vi "Map-characteristics.vi"(8 "error in (no error)":errorcluster, 11 "Data ref. in":refnum<data-value>) -> (0 "error out":errorcluster, 3 "Data ref.":refnum<data-value>)   [LabVIEW 2013, in "CameraVision.lvlib" / "CV-Main.lvclass"]
uses:
  CV-Main.lvclass
  Buffers/Mapping-buffer.ctl
  Temperature/Temperature-characteristics.ctl
  Analysis/Characteristics-cluster.ctl
  CV-Main.lvclass/CV-Main.ctl
  Buffers/CV-Buffers.lvclass/CV-Buffers.ctl
  Mapping/CV-Mapping.lvclass/CV-Mapping.ctl
  Read Buffers.vi
  Read Mapping params.vi
  Read Map.vi
  Read Processing.vi
  Mapping/Read Time.vi
  Mapping/Read Xcoors.vi
  Mapping/Read Ycoors.vi
  Mapping/Read Enable mapping.vi
  Buffers/Read Mapping buffer.vi
  Buffers/CV-Buffers.lvclass
  Mapping/CV-Mapping.lvclass
  UI/CV-UI.lvclass
  Temperature/CV-Temperature.lvclass
  Analysis/CV-Analysis.lvclass
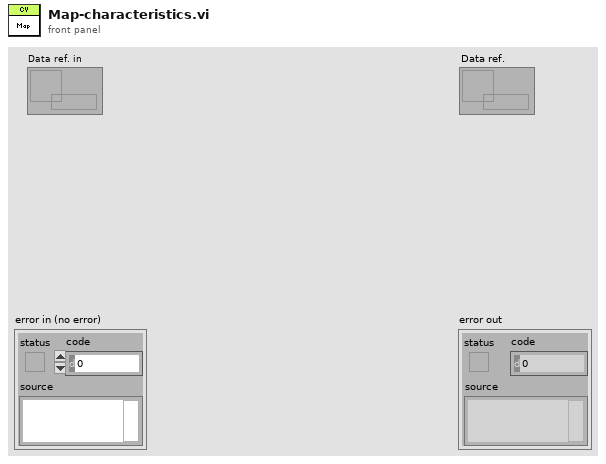
[diagram p1: front panel]
types:
  T1 = typedef "CameraVision.lvlib/CV-Buffers.lvclass/Mapping-buffer.ctl" = cluster{"Time":timestamp, "Index":i32, "Temperature characteristics":T2, "Characteristics":T3[], "Xcoord":sgl, "Ycoord":sgl}
  T2 = typedef "CameraVision.lvlib/CV-Temperature.lvclass/Temperature-characteristics.ctl" = cluster{"Average temperature ":dbl, "Max. temperature":dbl, "Min. temperature":dbl, "Stand. dev. temperature":dbl, "Datapoints":dbl}
  T3 = typedef "CameraVision.lvlib/CV-Analysis.lvclass/Characteristics-cluster.ctl" = cluster{"Average intensity":dbl, "Peak intensity":dbl, "Melt-pool size":dbl, "Melt-pool aspect ratio":dbl, "Melt-pool fragments":dbl, "Centre of mass X":dbl, "Centre of mass Y":dbl, "Orientation":dbl}
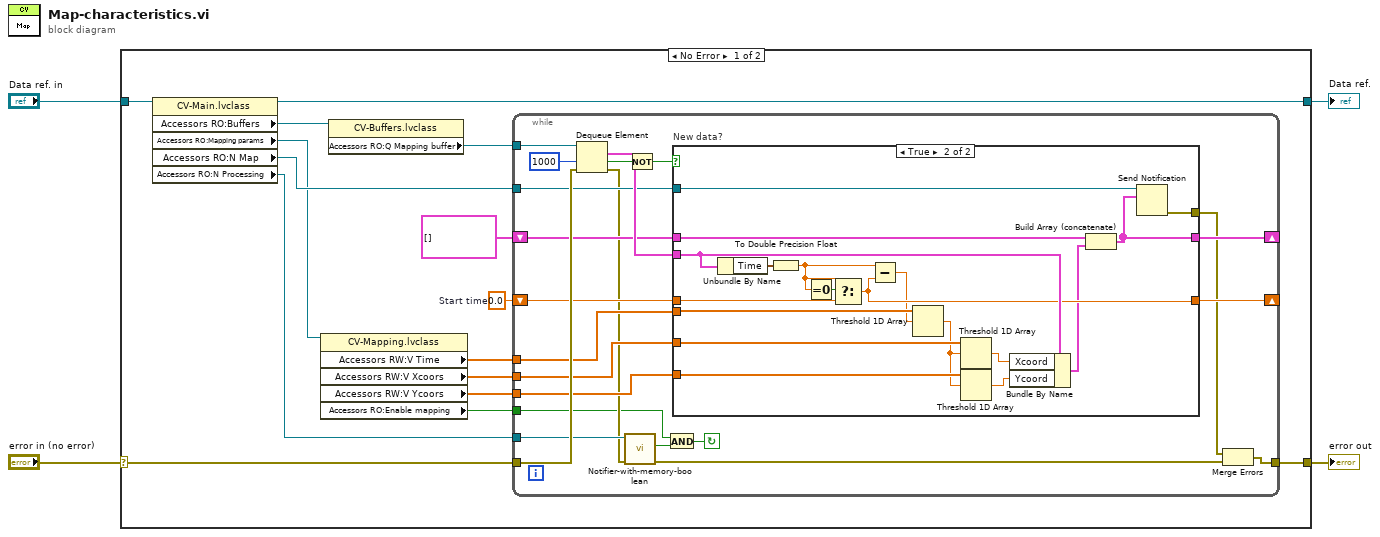
[diagram p0: block diagram]
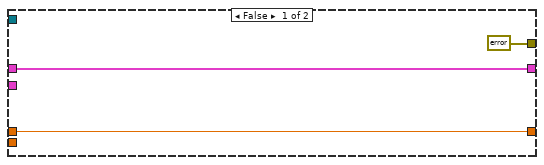
[diagram p2: hidden frame]
diagram:
  n1 = case shown="No Error" "error in (no error)" {
    selector: "error in (no error)" -> [w16 w64]
    tunnel: [w11 w64] -> w3
    tunnel: "Data ref. in" -> [w19 w63]
    tunnel: [w18 w63] -> w1
    frame No Error {
      w7 = 0.0  # Start time
      n2 = property class="CV-Main.lvclass"(reference=w19) -> (reference out=w18:refnum<data-value>, "Accessors RO:Buffers"=w17:refnum<class "CV-Buffers.lvclass">, "Accessors RO:Mapping params"=w12:refnum<data-value>, "Accessors RO:N Map"=w15:refnum<notifier>, "Accessors RO:N Processing"=w14:refnum<notifier>)  [unwired: 1 in, 1 out]
      n3 = property class="CV-Mapping.lvclass"(reference=w12) -> ("Accessors RW:V Time"=w10:sgl[], "Accessors RW:V Xcoors"=w9:sgl[], "Accessors RW:V Ycoors"=w8:sgl[], "Accessors RO:Enable mapping"=w5:bool)  [unwired: 1 in, 2 out]
      n4 = property class="CV-Buffers.lvclass"(reference=w17) -> ("Accessors RO:Q Mapping buffer"=w13:refnum<queue>)  [unwired: 1 in, 2 out]
      n5 = while {
        tunnel: w16 -> [w39]
        tunnel: w15 -> [w26]
        tunnel: w14 -> [w35]
        tunnel: w13 -> [w41]
        tunnel: [w25] -> w11
        tunnel: w10 -> [w34]
        tunnel: w9 -> [w33]
        tunnel: w8 -> [w32]
        shift-right: [w27] -> _
        shift-left: w7 -> [w28]
        shift-right: [w30] -> _
        shift-left: T1[] [] -> [w29]
        tunnel: w5 -> [w21]
        stop <- w20 continue-if-true
        n6 = Dequeue Element(queue=w41, timeout in ms (-1)=1000, error in (no error)=w39) -> (element=w31:T1, timed out?=w38:bool, error out=w23:errorcluster)  [unwired: 1 out]
        n7 = call "Notifier-with-memory-boolean.vi"("error in"=w23, "Notifier in"=w35) -> ("error IO"=w36:errorcluster, "Notification"=w22:bool)  [unwired: 8 in]
        n8 = Not(x=w38) -> (.not. x?=w37:bool)
        n9 = And(x=w21, y=w22) -> (x .and. y?=w20:bool)
        n10 = case "New data?" shown="True" w37 {
          tunnel: w34 -> [_ w55]
          tunnel: w33 -> [_ w53]
          tunnel: w32 -> [_ w52]
          tunnel: w31 -> [_ w59]
          tunnel: [w42 w45] -> w30
          tunnel: w29 -> [w42 w62]
          tunnel: w28 -> [w44 w60]
          tunnel: [w44 w56] -> w27
          tunnel: w26 -> [_ w47]
          tunnel: [errorcluster {"status"=FALSE, "code"=0, "source"=""} ("error out") w46] -> w24
          frame False {
          }
          frame True {
            n11 = Unbundle By Name(w59) -> ("Time"=w61:timestamp)
            n12 = To Double Precision Float(number=w61) -> (double precision float=w57:dbl)
            n13 = Equal To 0?(x=w57) -> (x = 0?=w58:bool)
            n14 = Select(t=w57, s=w58, f=w60) -> (s? t:f=w56:dbl)
            n15 = Subtract(x=w57, y=w56) -> (x-y=w54:dbl)
            n16 = Threshold 1D Array(2:w54, 3:w55) -> (0:w51:sgl)  [unwired: 1 in]
            n17 = Threshold 1D Array(2:w51, 3:w53) -> (0:w48:sgl)  [unwired: 1 in]
            n18 = Threshold 1D Array(2:w51, 3:w52) -> (0:w49:sgl)  [unwired: 1 in]
            n19 = Bundle By Name(cluster=w59, "Xcoord"=w48, "Ycoord"=w49) -> (w50:T1)
            n20 = Build Array (concatenate)(w62, w50) -> (w45:T1[])
            n21 = Send Notification(notification=w45, notifier=w47) -> (error out=w46:errorcluster)  [unwired: 1 in, 1 out]
          }
        }
        n22 = Merge Errors(w24, w36) -> (w25:errorcluster)
      }
    }
    frame Error {
    }
  }
  "error out" <- w3
  "Data ref." <- w1
